vi "GT Buf Event On.vi"(6 "fifo":i16, 7 "count":i16, 8 "error in (no error)":errorcluster caption="错误输入（无错误）", 9 "eventIndex":i16, 10 "crd":i16, 11 "cardNum":i16) -> (0 "error out":errorcluster caption="错误输出", 3 "cardNum":i16)   [LabVIEW 2020, in "gts1.lvlib"]
doc: "GT_API GT_BufEventOn(short cardNum,short crd,short eventIndex,short count,short fifo);"
uses:
  gts1.lvlib
  dll/32bit/multi_card/gts.dll
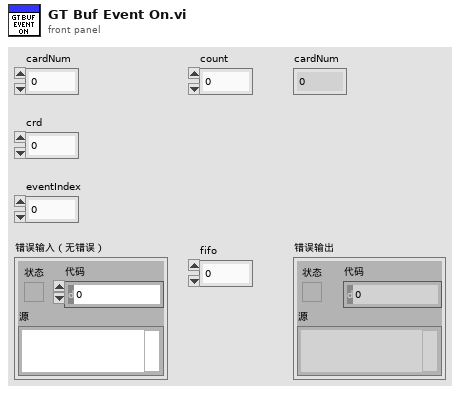
[diagram p1: front panel]
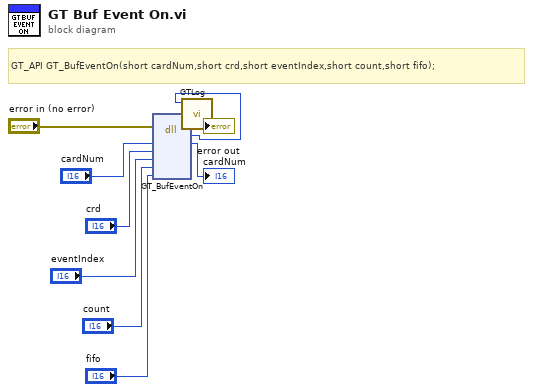
[diagram p0: block diagram]
diagram:
  # "GT_API GT_BufEventOn(short cardNum,short crd,short eventIndex,short count,short fifo);"
  n1 = dll-call lib="D:/Git/GoogolCard/dll/32bit/multi_card/gts.dll" fn="GT_BufEventOn"(error in="error in (no error)", "cardNum"="cardNum", "crd"="crd", "eventIndex"="eventIndex", "count"="count", "fifo"="fifo") -> (error out=w4:errorcluster, w2:i16, "cardNum"=→"cardNum":i16)  [unwired: 6 in, 1 out]
  n2 = call "GTLog.vi"("error in (no error)"=w4, "Numeric"=w2) -> ("error out"=→"error out":errorcluster)  [unwired: 9 in]
